vi "Turn Right.vi"(6 "Turning angle":sgl=45.0, 7 "Motor":cluster{"Port":T2, "Port":T2}={"Port"=1, "Port"=2} {"Port" items=["Port A", "Port B", "Port C", "Port D"]; "Port" items=["Port A", "Port B", "Port C", "Port D"]}, 10 "Motor B (right)":i8=50, 11 "EV3 in":T1) -> (3 "EV3 out":T1)   [LabVIEW 2016]
uses:
  <vilib>/NXT/Block Support/NXT_OutputPort.ctl
  <vilib>/NXT/Subs/LVHSConnector.ctl
  <vilib>/NXT/LegoClasses/BrickReference/BrickReference.lvclass
  <vilib>/NXT/Block Support/NXT_InputPort.ctl
  <vilib>/NXT/NXTIO Xnodes/NXTIONodeSubVIs/NXTMoveMotors.vi
  <vilib>/NXT/Dual Mode Library/Sensors/EV3_Gyro_Angle.vi
  <vilib>/NXT/NXTIO Xnodes/NXTIONodeSubVIs/NXTStopMotors.vi
  <vilib>/NXT/NXTIO Xnodes/NXTIONodeSubVIs/LEGOResetMotors.vi
  <vilib>/NXT/Dual Mode Library/Waits/Wait_Num.vi
  <vilib>/NXT/NXTIO Xnodes/NXTIOXNode/NXTIO.xnode
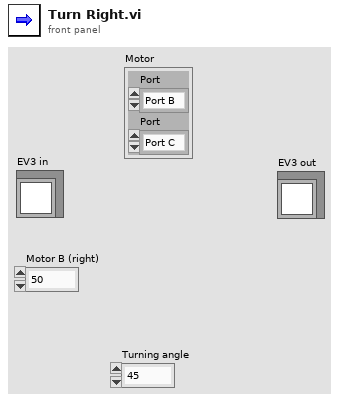
[diagram p1: front panel]
types:
  T1 = typedef "LVHSConnector.ctl" = refnum<class "BrickReference.lvclass">
  T2 = typedef "NXT_OutputPort.ctl" = u8
  T3 = typedef "NXT_InputPort.ctl" = u32
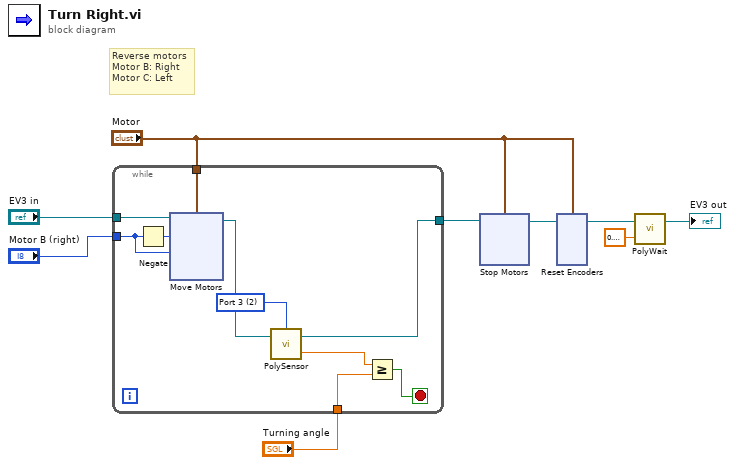
[diagram p0: block diagram]
diagram:
  # "Reverse motors\nMotor B: Right\nMotor C: Left"
  n1 = while {
    tunnel: [w15] -> w6
    tunnel: "EV3 in" -> [w14]
    tunnel: "Motor" -> [w13]
    tunnel: "Turning angle" -> [w12]
    tunnel: "Motor B (right)" -> [w10]
    stop <- w18 stop-if-true
    w17 = T3 2 items=["Port 1", "Port 2", "Port 3", "Port 4"] ("Port (Port 1)")
    n2 = Negate(x=w10) -> (-x=w11:i8)
    n3 = xnode "Move Motors"("Power/Speed 2"=w10, "Power/Speed 1"=w11, "Motors"=w13, "NXT/EV3"=w14) -> ("NXT/EV3"=w16:T1)
    n4 = call-poly <vilib>:"PolySensor.vi"("NXT/EV3"=w16, "Port (Port 1)"=w17) -> ("Degrees"=w19:sgl, "NXT/EV3"=w15:T1)  [unwired: 1 in]
    n5 = Greater Or Equal?(x=w19, y=w12) -> (x >= y?=w18:bool)
  }
  n6 = xnode "Stop Motors"("Motors"="Motor", "NXT/EV3"=w6) -> ("NXT/EV3"=w5:T1)
  n7 = xnode "Reset Encoders"("Motors"="Motor", "NXT/EV3"=w5) -> ("NXT/EV3"=w2:T1)
  n8 = call-poly <vilib>:"PolyWait.vi"("Time (1 sec)"=sgl 0.2, "NXT/EV3"=w2) -> ("NXT/EV3"=→"EV3 out":T1)  [unwired: 2 in]
